vi "DataTreeCtrl saveAsMAT.vi"(8 "error in (no error)":errorcluster, 11 "DataTreeCtrl in":refnum<class "DataTreeCtrl.lvclass">) -> (0 "error out":errorcluster, 3 "DataTreeCtrl out":refnum<class "DataTreeCtrl.lvclass">)   [LabVIEW 2018, in "DataTreeCtrl.lvclass"]
uses:
  DataTreeCtrl.lvclass
  ctl/FMstateMachineEnum.ctl
  DataTreeCtrl.lvclass/DataTreeCtrl.ctl
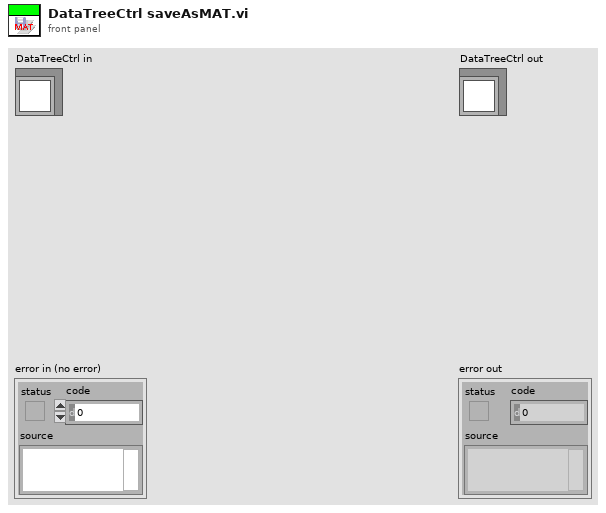
[diagram p1: front panel]
types:
  T1 = enum16{"open", "open or create", "create or replace", "create", "open (read only)"}
  T2 = typedef "FMstateMachineEnum.ctl" = enum16{"none", "init", "openTDMS", "closeTDMS", "getDataList", "getDataInfo", "getTimeStamp", "getCurrPath", "getRemark", "overwriteRemark", "readData", "deleteData", "moveData"}
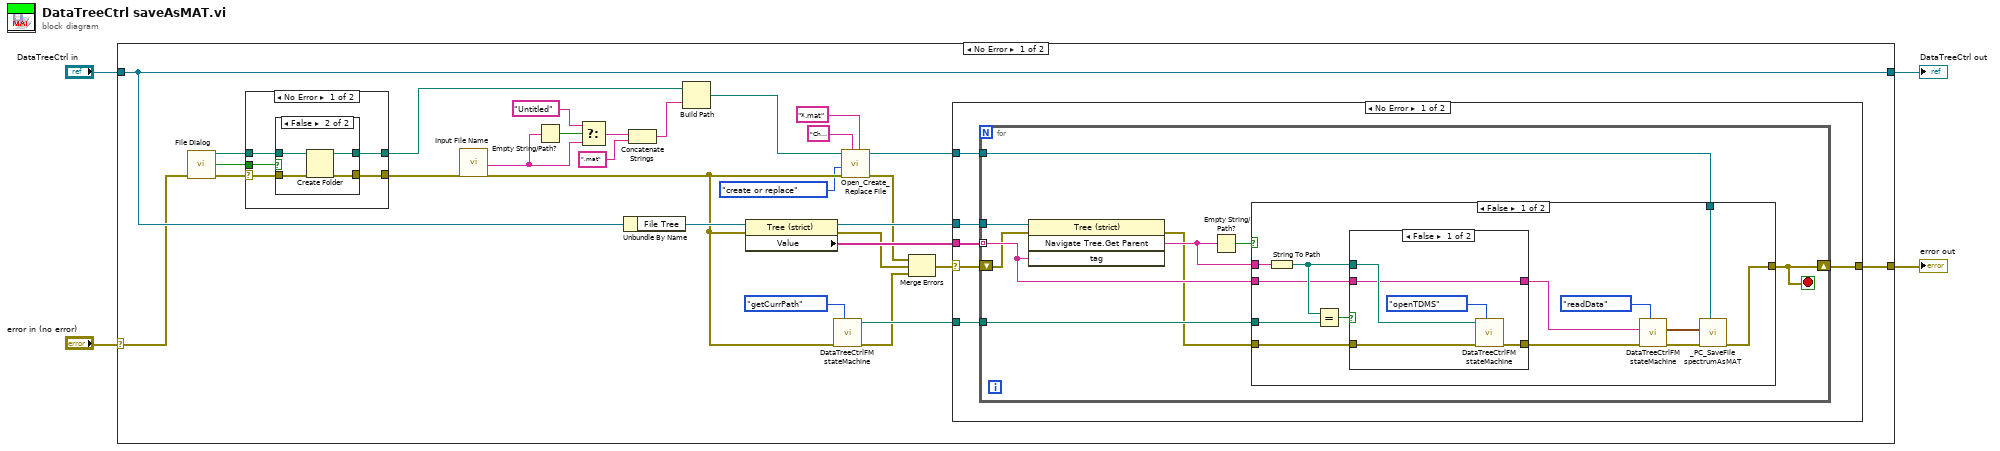
[diagram p0: block diagram]
diagram:
  n1 = case shown="No Error" "error in (no error)" {
    selector: "error in (no error)" -> [w24 w85]
    tunnel: [w6 w85] -> w3
    tunnel: [w32 w84] -> w1
    tunnel: "DataTreeCtrl in" -> [w32 w84]
    frame No Error {
      n2 = call "File Dialog"("error in"=w24) -> ("selected path"=w27:path, "exists"=w26:bool, "error out"=w25:errorcluster)  [unwired: 11 in, 1 out]
      n3 = case shown="No Error" w25 {
        selector: w25 -> [w73 w83]
        tunnel: w26 -> [w75 _]
        tunnel: w27 -> [w74 w82]
        tunnel: [w72 w83] -> w12
        tunnel: [w71 w82] -> w18
        frame No Error {
          n4 = case shown="False" w75 {
            tunnel: w74 -> [w76 w81]
            tunnel: w73 -> [w77 w80]
            tunnel: [w77 w79] -> w72
            tunnel: [w76 w78] -> w71
            frame True {
            }
            frame False {
              n5 = Create Folder(path (use dialog)=w81, error in=w80) -> (created path=w78:path, error out=w79:errorcluster)  [unwired: 1 in, 1 out]
            }
          }
        }
        frame Error {
        }
      }
      n6 = call "Input File Name"("error in (no error)"=w12) -> ("file name"=w23:string, "error out"=w8:errorcluster)  [unwired: 16 in, 1 out]
      n7 = Empty String/Path?(string/path=w23) -> (empty?=w22:bool)
      n8 = Select(t="Untitled", s=w22, f=w23) -> (s? t:f=w19:string)
      n9 = Unbundle By Name(w32) -> ("File Tree"=w33:refnum<vi>)
      n10 = Concatenate Strings(w19, ".mat" ("pattern")) -> (w17:string)
      n11 = Build Path(base path=w18, name or relative path=w17) -> (appended path=w14:path)
      n12 = property class="Tree (strict)"(reference=w33, error in=w8) -> (reference out=w29:refnum<vi>, error out=w10:errorcluster, "Value"=w30:string[])
      n13 = call "DataTreeCtrlFM stateMachine.vi"("Func"=FMstateMachineEnum."getCurrPath", "error in (no error)"=w8) -> ("error out"=w9:errorcluster, "tdmsFilePath out"=w28:path)  [unwired: 4 in, 4 out]
      n14 = call <vilib>:"Open_Create_Replace File.vi"("pattern"="*.mat", "prompt"="Choose new or existing MATLAB data file", "error in (no error)"=w8, "function (open:0)"=T1."create or replace", "file path"=w14) -> ("error out"=w11:errorcluster, "refnum"=w13:refnum<file>)  [unwired: 3 in, 2 out]
      n15 = Merge Errors(w11, w10, w9) -> (w7:errorcluster)
      n16 = case shown="No Error" w7 {
        selector: w7 -> [w35 w70]
        tunnel: w30 -> [w39 _]
        tunnel: w29 -> [w38 _]
        tunnel: w28 -> [w37 _]
        tunnel: w13 -> [w36 _]
        tunnel: [w34 w70] -> w6
        frame No Error {
          n17 = for {
            tunnel: w39 -> [w48] mode=indexing
            tunnel: w38 -> [w47]
            tunnel: w37 -> [w46]
            tunnel: w36 -> [w45]
            shift-right: [w40] -> w34
            shift-left: w35 -> [w44]
            stop <- w40 stop-if-true
            n18 = invoke class="Tree (strict)" method="Navigate Tree.Get Parent"(reference=w47, error in=w44, "tag"=w48) -> (error out=w41:errorcluster, "Navigate Tree:Get Parent"=w42:string)  [unwired: 1 in, 2 out]
            n19 = Empty String/Path?(string/path=w42) -> (empty?=w43:bool)
            n20 = case shown="False" w43 {
              tunnel: w42 -> [w61 _]
              tunnel: w46 -> [w60 _]
              tunnel: w48 -> [w58 _]
              tunnel: w41 -> [w56 w69]
              tunnel: w45 -> [w50 _]
              tunnel: [w49 w69] -> w40
              frame False {
                n21 = String To Path(string=w61) -> (path=w59:path)
                n22 = Equal?(x=w59, y=w60) -> (x = y?=w57:bool)
                n23 = case shown="False" w57 {
                  tunnel: w58 -> [w62 w67]
                  tunnel: w56 -> [w64 w68]
                  tunnel: [w63 w68] -> w54
                  tunnel: w59 -> [w65 _]
                  tunnel: [w62 w67] -> w53
                  frame False {
                    n24 = call "DataTreeCtrlFM stateMachine.vi"("Func"=FMstateMachineEnum."openTDMS", "error in (no error)"=w64, "tdmsFilePath in"=w65) -> ("error out"=w63:errorcluster)  [unwired: 3 in, 5 out]
                  }
                  frame True {
                  }
                }
                n25 = call "DataTreeCtrlFM stateMachine.vi"("Func"=FMstateMachineEnum."readData", "error in (no error)"=w54, "singleDataName"=w53) -> ("error out"=w51:errorcluster, "signalData"=w52:waveform(sgl))  [unwired: 3 in, 4 out]
                n26 = call "_PC_SaveFile spectrumAsMAT.vi"("path refnum in"=w50, "error in (no error)"=w51, "Spectrum data in"=w52) -> ("error out"=w49:errorcluster)  [unwired: 8 in]
              }
              frame True {
              }
            }
          }
        }
        frame Error {
        }
      }
    }
    frame Error {
    }
  }
  "error out" <- w3
  "DataTreeCtrl out" <- w1
